vi "Connect.vi"(8 "error in (no error)":errorcluster, 9 "Default Headers":T1(array[cluster]), 10 "Authentication":cluster{"Username":string, "Password":string}, 11 "REST Interface in":refnum<class "EnVision REST.lvclass">) -> (0 "error out":errorcluster, 3 "REST Interface out":refnum<class "EnVision REST.lvclass">)   [LabVIEW 2018, in "EnVision REST.lvlib" / "EnVision REST.lvclass"]
uses:
  EnVision REST.lvclass
  EnVision REST.lvclass/EnVision REST.ctl
  PPLs/REST Interface/Parent/REST Interface.lvlibp/REST Interface.lvclass
  <vilib>/addons/_JKI.lib/REST Client/classes/REST Client/REST Client.lvclass
  C:/Projects/LabVIEW/PPLs/REST Interface/Parent/REST Interface.lvlibp/REST Interface.lvclass
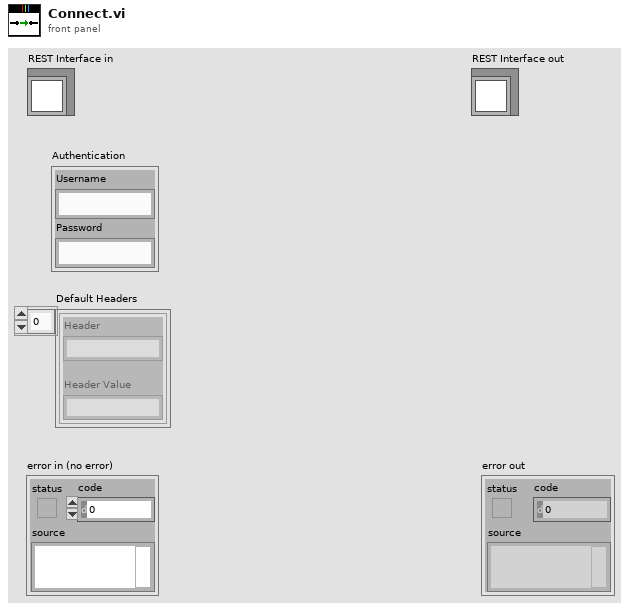
[diagram p1: front panel]
types:
  T1 = cluster{"Header":string, "Header Value":string}[]
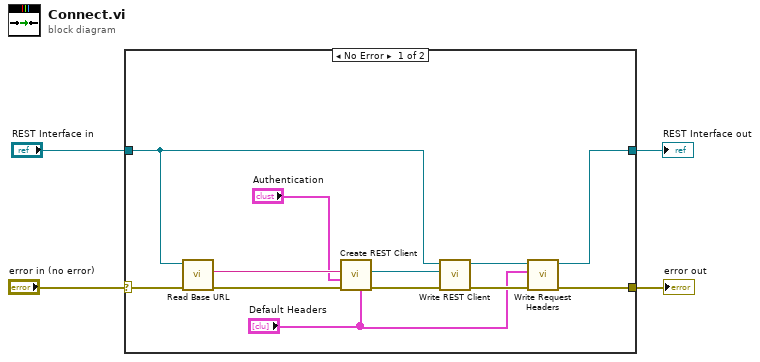
[diagram p0: block diagram]
diagram:
  n1 = case shown="No Error" "error in (no error)" {
    selector: "error in (no error)" -> [w16 w18]
    tunnel: [w6 w18] -> w3
    tunnel: [w7 w17] -> w2
    tunnel: "REST Interface in" -> [w10 w17]
    frame No Error {
      n2 = call "Read Base URL.vi"("error in (no error)"=w16, "REST Interface in"=w10) -> ("error out"=w14:errorcluster, "Base URL"=w15:string)  [unwired: 7 in, 1 out]
      n3 = call <vilib>:"Create REST Client.vi"("Default Headers ([JSON])"="Default Headers", "error in (no error)"=w14, "Authentication"="Authentication", "Base URL"=w15) -> ("error out"=w12:errorcluster, "REST Client out"=w13:refnum<class "REST Client.lvclass">)  [unwired: 6 in]
      n4 = call "Write REST Client.vi"("error in (no error)"=w12, "REST Client.lvlib:REST Client.lvclass"=w13, "EnVision REST in"=w10) -> ("error out"=w9:errorcluster, "EnVision REST out"=w8:refnum<class "EnVision REST.lvclass">)  [unwired: 7 in]
      n5 = call "Write Request Headers.vi"("error in (no error)"=w9, "Request Headers"="Default Headers", "REST Interface in"=w8) -> ("error out"=w6:errorcluster, "REST Interface out"=w7:refnum<class "EnVision REST.lvclass">)  [unwired: 7 in]
    }
    frame Error {
    }
  }
  "error out" <- w3
  "REST Interface out" <- w2
